vi "I(V)_K6221-K2182a_PK_fixedrange.vi"() -> ()   [LabVIEW 2016]
uses:
  Labview Drivers/Keithley 622x LV 2009/Configure/Source/Typedefs/KE622x -- Current Range.ctl
  Labview Drivers/Keithley 622x LV 2009/Configure/Source/Typedefs/KE622x -- Current Ranges.ctl
  Labview Drivers/Keithley 622x LV 2009/Keithley 622x.lvlib
panel:
  in  "Current Range In":T1
  out "Resistance (ohm)":dbl=inf format="%#_13g"
  out "Time (s)":dbl=95.61940909968689 format="%#_13g"
  in  "Total number of I-V loops":i32=1
  in  "Numeric Average":i32=1
  in  "wait (ms)":u32=50
  out "Iset (A)":dbl
  out "Vmeas (V)":dbl=1.84890386e-07
  in  "Folder":path=path "D:/Pranava/Data/PtTe2/31-05-2022/001/after warmup"
  in  "Set Compliance voltage (V)":dbl=20.0 min=0.0 step=0.1 format="%_3f"
  out "I vs V":cluster{dbl, "Field Reading":dbl}[](graph)=[{0.0, "Field Reading"=5.69524003e-09}, {1e-06, "Field Reading"=1.86435146e-08}, {2e-06, "Field Reading"=-1.55399303e-08}, {3e-06, "Field Reading"=5.69524003e-09}, {4e-06, "Field Reading"=1.03168822e-09}, {5e-06, "Field Reading"=-4.50641504e-08}, {6e-06, "Field Reading"=1.9677196e-08}, {7e-06, "Field Reading"=2.48565037e-08}, {8e-06, "Field Reading"=-4.71358735e-08}, {9e-06, "Field Reading"=3.52151191e-08}, {1e-05, "Field Reading"=1.08723729e-08}, {1.1e-05, "Field Reading"=1.34588038e-08}, {1.2e-05, "Field Reading"=-8.8122059e-09}, {1.3e-05, "Field Reading"=-8.8122059e-09}, {1.4e-05, "Field Reading"=3.00325784e-08}, {1.5e-05, "Field Reading"=1.08691515e-08}, {1.6e-05, "Field Reading"=3.10019462e-09}, {1.7e-05, "Field Reading"=-4.66876224e-09}, {1.8e-05, "Field Reading"=2.38174129e-08}, {1.9e-05, "Field Reading"=2.58874074e-08}, {2e-05, "Field Reading"=-2.90132033e-08}, {2.1e-05, "Field Reading"=-1.7618737e-08}, {2.2e-05, "Field Reading"=5.43735733e-08}, {2.3e-05, "Field Reading"=-3.05669942e-08}, {2.4e-05, "Field Reading"=4.76404796e-08}, {2.5e-05, "Field Reading"=-2.4869761e-08}, {2.6e-05, "Field Reading"=1.34592487e-08}, {2.7e-05, "Field Reading"=-5.70417987e-09}, {2.8e-05, "Field Reading"=-5.17999945e-08}, {2.9e-05, "Field Reading"=3.31406077e-08}, {3e-05, "Field Reading"=-3.41903574e-08}, {3.1e-05, "Field Reading"=4.29812872e-08}, {3.2e-05, "Field Reading"=2.17461367e-08}, {3.3e-05, "Field Reading"=1.54751787e-09}, {3.4e-05, "Field Reading"=-1.34724686e-08}, {3.5e-05, "Field Reading"=1.13881986e-08}, {3.6e-05, "Field Reading"=-4.19586497e-08}, {3.7e-05, "Field Reading"=2.27826711e-08}, {3.8e-05, "Field Reading"=-8.29316289e-09}, {3.9e-05, "Field Reading"=1.54751787e-09}, {4e-05, "Field Reading"=-5.70351006e-09}, {4.1e-05, "Field Reading"=-1.70968827e-08}, {4.2e-05, "Field Reading"=1.0353443e-08}, {4.3e-05, "Field Reading"=4.35010061e-08}, {4.4e-05, "Field Reading"=1.91582645e-08}, {4.5e-05, "Field Reading"=-3.05630803e-08}, {4.6e-05, "Field Reading"=-4.97265152e-08}, {4.7e-05, "Field Reading"=1.81224031e-08}, {4.8e-05, "Field Reading"=-2.64182465e-08}, {4.9e-05, "Field Reading"=-2.17568692e-08}, {5e-05, "Field Reading"=-2.17568692e-08}, {5.1e-05, "Field Reading"=-2.7972039e-08}, {5.2e-05, "Field Reading"=2.79644885e-08}, {5.3e-05, "Field Reading"=9.31897937e-09}, {5.4e-05, "Field Reading"=2.38210421e-08}, {5.5e-05, "Field Reading"=-1.0884604e-08}, {5.6e-05, "Field Reading"=4.24622263e-08}, {5.7e-05, "Field Reading"=3.09951655e-09}, {5.8e-05, "Field Reading"=-9.84874324e-09}, {5.9e-05, "Field Reading"=-4.14424971e-08}, {6e-05, "Field Reading"=4.8677391e-08}, {6.1e-05, "Field Reading"=6.11077204e-08}, {6.2e-05, "Field Reading"=1.13864028e-08}, {6.3e-05, "Field Reading"=-1.86539399e-08}, {6.4e-05, "Field Reading"=2.34902041e-05}, {6.5e-05, "Field Reading"=2.39584131e-05}, {6.6e-05, "Field Reading"=2.43251077e-05}, {6.7e-05, "Field Reading"=2.47192527e-05}, {6.8e-05, "Field Reading"=2.51320432e-05}, {6.9e-05, "Field Reading"=2.55598536e-05}, {7e-05, "Field Reading"=2.60389398e-05}, {7.1e-05, "Field Reading"=2.63802559e-05}, {7.2e-05, "Field Reading"=2.6751612e-05}, {7.3e-05, "Field Reading"=2.72110162e-05}, {7.4e-05, "Field Reading"=2.76004998e-05}, {7.5e-05, "Field Reading"=2.79930909e-05}, {7.6e-05, "Field Reading"=2.83862001e-05}, {7.7e-05, "Field Reading"=2.87430612e-05}, {7.8e-05, "Field Reading"=2.92268082e-05}, {7.9e-05, "Field Reading"=2.95531044e-05}, {8e-05, "Field Reading"=2.99746998e-05}, {8.1e-05, "Field Reading"=3.04107972e-05}, {8.2e-05, "Field Reading"=3.08132291e-05}, {8.3e-05, "Field Reading"=3.1164386e-05}, {8.4e-05, "Field Reading"=3.15694075e-05}, {8.5e-05, "Field Reading"=3.20283147e-05}, {8.6e-05, "Field Reading"=3.24348904e-05}, {8.7e-05, "Field Reading"=3.27865653e-05}, {8.8e-05, "Field Reading"=3.32169657e-05}, {8.9e-05, "Field Reading"=3.36380434e-05}, {9e-05, "Field Reading"=3.39819494e-05}, {9.1e-05, "Field Reading"=3.44465424e-05}, {9.2e-05, "Field Reading"=3.48645126e-05}, {9.3e-05, "Field Reading"=3.52482993e-05}, {9.4e-05, "Field Reading"=3.5625353e-05}, {9.5e-05, "Field Reading"=3.60288211e-05}, {9.6e-05, "Field Reading"=3.64131257e-05}, {9.7e-05, "Field Reading"=3.68409366e-05}, {9.8e-05, "Field Reading"=3.72257592e-05}, {9.9e-05, "Field Reading"=3.76105824e-05}, {0.0001, "Field Reading"=3.80508236e-05}, {0.000101, "Field Reading"=3.84517021e-05}, {0.000102, "Field Reading"=3.87945723e-05}, {0.000103, "Field Reading"=3.92016659e-05}, {0.000104, "Field Reading"=3.96232616e-05}, {0.000105, "Field Reading"=4.00904352e-05}, {0.000106, "Field Reading"=4.04229382e-05}, {0.000107, "Field Reading"=4.09087573e-05}, {0.000108, "Field Reading"=4.12573246e-05}, {0.000109, "Field Reading"=4.16566492e-05}, {0.00011, "Field Reading"=4.20709938e-05}, {0.000111, "Field Reading"=4.24951791e-05}, {0.000112, "Field Reading"=4.28644637e-05}, {0.000113, "Field Reading"=4.32772566e-05}, {0.000114, "Field Reading"=4.3693155e-05}, {0.000115, "Field Reading"=4.41230375e-05}, {0.000116, "Field Reading"=4.44912863e-05}, {0.000117, "Field Reading"=4.4905113e-05}, {0.000118, "Field Reading"=4.53142783e-05}, {0.000119, "Field Reading"=4.57451966e-05}, {0.00012, "Field Reading"=4.61693819e-05}, {0.000121, "Field Reading"=4.65593711e-05}, {0.000122, "Field Reading"=4.69462653e-05}, {0.000123, "Field Reading"=4.74134387e-05}, {0.000124, "Field Reading"=4.78179425e-05}, {0.000125, "Field Reading"=4.81789402e-05}, {0.000126, "Field Reading"=4.86310936e-05}, {0.000127, "Field Reading"=4.90894622e-05}, {0.000128, "Field Reading"=4.94913942e-05}, {0.000129, "Field Reading"=4.98182085e-05}, {0.00013, "Field Reading"=5.02667366e-05}, {0.000131, "Field Reading"=5.07411612e-05}, {0.000132, "Field Reading"=5.11741513e-05}, {0.000133, "Field Reading"=5.15320415e-05}, {0.000134, "Field Reading"=5.1924633e-05}, {0.000135, "Field Reading"=5.22545517e-05}, {0.000136, "Field Reading"=5.27786976e-05}, {0.000137, "Field Reading"=5.32028829e-05}, {0.000138, "Field Reading"=5.35498965e-05}, {0.000139, "Field Reading"=5.39668308e-05}, {0.00014, "Field Reading"=5.44692236e-05}, {0.000141, "Field Reading"=5.47851614e-05}, {0.000142, "Field Reading"=5.52129722e-05}, {0.000143, "Field Reading"=5.56153793e-05}, {0.000144, "Field Reading"=5.60509589e-05}, {0.000145, "Field Reading"=5.64575344e-05}, {0.000146, "Field Reading"=5.68423568e-05}, {0.000147, "Field Reading"=5.7332837e-05}, {0.000148, "Field Reading"=5.77010856e-05}, {0.000149, "Field Reading"=5.80838363e-05}, {0.00015, "Field Reading"=5.85660081e-05}, {0.00015, "Field Reading"=5.85986377e-05}, {0.000149, "Field Reading"=5.80952094e-05}, {0.000148, "Field Reading"=5.767465e-05}, {0.000147, "Field Reading"=5.73058836e-05}, {0.000146, "Field Reading"=5.68801448e-05}, {0.000145, "Field Reading"=5.65103425e-05}, {0.000144, "Field Reading"=5.60778901e-05}, {0.000143, "Field Reading"=5.56329878e-05}, {0.000142, "Field Reading"=5.52310737e-05}, {0.000141, "Field Reading"=5.48478051e-05}, {0.00014, "Field Reading"=5.43966876e-05}, {0.000139, "Field Reading"=5.39958094e-05}, {0.000138, "Field Reading"=5.36083974e-05}, {0.000137, "Field Reading"=5.31334551e-05}, {0.000136, "Field Reading"=5.27263627e-05}, {0.000135, "Field Reading"=5.23539706e-05}, {0.000134, "Field Reading"=5.19701841e-05}, {0.000133, "Field Reading"=5.15102618e-05}, {0.000132, "Field Reading"=5.10767539e-05}, {0.000131, "Field Reading"=5.06815729e-05}, {0.00013, "Field Reading"=5.03112526e-05}, {0.000129, "Field Reading"=4.99316069e-05}, {0.000128, "Field Reading"=4.95022425e-05}, {0.000127, "Field Reading"=4.90236747e-05}, {0.000126, "Field Reading"=4.86590516e-05}, {0.000125, "Field Reading"=4.8298054e-05}, {0.000124, "Field Reading"=4.78526338e-05}, {0.000123, "Field Reading"=4.74331101e-05}, {0.000122, "Field Reading"=4.70338163e-05}, {0.000121, "Field Reading"=4.66567626e-05}, {0.00012, "Field Reading"=4.62491511e-05}, {0.000119, "Field Reading"=4.58311809e-05}, {0.000118, "Field Reading"=4.54318562e-05}, {0.000117, "Field Reading"=4.50506591e-05}, {0.000116, "Field Reading"=4.45938441e-05}, {0.000115, "Field Reading"=4.41727664e-05}, {0.000114, "Field Reading"=4.37987887e-05}, {0.000113, "Field Reading"=4.34227711e-05}, {0.000112, "Field Reading"=4.29882274e-05}, {0.000111, "Field Reading"=4.25780265e-05}, {0.00011, "Field Reading"=4.22341206e-05}, {0.000109, "Field Reading"=4.18316886e-05}, {0.000108, "Field Reading"=4.13986987e-05}, {0.000107, "Field Reading"=4.09154706e-05}, {0.000106, "Field Reading"=4.05446324e-05}, {0.000105, "Field Reading"=4.01655073e-05}, {0.000104, "Field Reading"=3.97755056e-05}, {0.000103, "Field Reading"=3.94046673e-05}, {0.000102, "Field Reading"=3.89846257e-05}, {0.000101, "Field Reading"=3.85687275e-05}, {0.0001, "Field Reading"=3.81668178e-05}, {9.9e-05, "Field Reading"=3.77840672e-05}, {9.8e-05, "Field Reading"=3.73800813e-05}, {9.7e-05, "Field Reading"=3.6964701e-05}, {9.6e-05, "Field Reading"=3.65876475e-05}, {9.5e-05, "Field Reading"=3.61862513e-05}, {9.4e-05, "Field Reading"=3.57418669e-05}, {9.3e-05, "Field Reading"=3.54010586e-05}, {9.2e-05, "Field Reading"=3.49520129e-05}, {9.1e-05, "Field Reading"=3.45050389e-05}, {9e-05, "Field Reading"=3.41409338e-05}, {8.9e-05, "Field Reading"=3.37934025e-05}, {8.8e-05, "Field Reading"=3.33686995e-05}, {8.7e-05, "Field Reading"=3.2970411e-05}, {8.6e-05, "Field Reading"=3.2593365e-05}, {8.5e-05, "Field Reading"=3.22489412e-05}, {8.4e-05, "Field Reading"=3.17481023e-05}, {8.3e-05, "Field Reading"=3.14010889e-05}, {8.2e-05, "Field Reading"=3.09567045e-05}, {8.1e-05, "Field Reading"=3.05817227e-05}, {8e-05, "Field Reading"=3.01492507e-05}, {7.9e-05, "Field Reading"=2.97685718e-05}, {7.8e-05, "Field Reading"=2.93438618e-05}, {7.7e-05, "Field Reading"=2.90129043e-05}, {7.6e-05, "Field Reading"=2.85358903e-05}, {7.5e-05, "Field Reading"=2.81464066e-05}, {7.4e-05, "Field Reading"=2.78107877e-05}, {7.3e-05, "Field Reading"=2.73721006e-05}, {7.2e-05, "Field Reading"=2.69810631e-05}, {7.1e-05, "Field Reading"=2.6545994e-05}, {7e-05, "Field Reading"=2.61259525e-05}, {6.9e-05, "Field Reading"=2.5727664e-05}, {6.8e-05, "Field Reading"=2.54143162e-05}, {6.7e-05, "Field Reading"=2.49150313e-05}, {6.6e-05, "Field Reading"=2.45364243e-05}, {6.5e-05, "Field Reading"=2.41101676e-05}, {6.4e-05, "Field Reading"=2.37274173e-05}, {6.3e-05, "Field Reading"=2.32561007e-05}, {6.2e-05, "Field Reading"=2.28702426e-05}, {6.1e-05, "Field Reading"=2.24574521e-05}, {6e-05, "Field Reading"=2.20229085e-05}, {5.9e-05, "Field Reading"=2.15950981e-05}, {5.8e-05, "Field Reading"=2.11512318e-05}, {5.7e-05, "Field Reading"=2.07586406e-05}, {5.6e-05, "Field Reading"=2.03329035e-05}, {5.5e-05, "Field Reading"=1.98952523e-05}, {5.4e-05, "Field Reading"=1.94612267e-05}, {5.3e-05, "Field Reading"=1.90038942e-05}, {5.2e-05, "Field Reading"=1.8551223e-05}, {5.1e-05, "Field Reading"=1.80809422e-05}, {5e-05, "Field Reading"=1.76241276e-05}, {4.9e-05, "Field Reading"=1.71724962e-05}, {4.8e-05, "Field Reading"=1.66587092e-05}, {4.7e-05, "Field Reading"=1.61713366e-05}, {4.6e-05, "Field Reading"=1.56368323e-05}, {4.5e-05, "Field Reading"=1.51396191e-05}, {4.4e-05, "Field Reading"=1.45895769e-05}, {4.3e-05, "Field Reading"=1.40100127e-05}, {4.2e-05, "Field Reading"=1.33589784e-05}, {4.1e-05, "Field Reading"=1.27302107e-05}, {4e-05, "Field Reading"=1.20978174e-05}, {3.9e-05, "Field Reading"=1.13219574e-05}, {3.8e-05, "Field Reading"=1.03239051e-05}, {3.7e-05, "Field Reading"=9.26473704e-06}, {3.6e-05, "Field Reading"=2.63103012e-07}, {3.5e-05, "Field Reading"=2.08202367e-07}, {3.4e-05, "Field Reading"=2.38242436e-07}, {3.3e-05, "Field Reading"=2.5015484e-07}, {3.2e-05, "Field Reading"=2.13899697e-07}, {3.1e-05, "Field Reading"=2.51708632e-07}, {3e-05, "Field Reading"=1.90074888e-07}, {2.9e-05, "Field Reading"=2.22704517e-07}, {2.8e-05, "Field Reading"=2.64656898e-07}, {2.7e-05, "Field Reading"=2.52744229e-07}, {2.6e-05, "Field Reading"=2.12863572e-07}, {2.5e-05, "Field Reading"=2.82784203e-07}, {2.4e-05, "Field Reading"=1.75054638e-07}, {2.3e-05, "Field Reading"=1.94736001e-07}, {2.2e-05, "Field Reading"=2.50672506e-07}, {2.1e-05, "Field Reading"=2.7138973e-07}, {2e-05, "Field Reading"=2.04059697e-07}, {1.9e-05, "Field Reading"=2.51709321e-07}, {1.8e-05, "Field Reading"=2.38761053e-07}, {1.7e-05, "Field Reading"=2.59478281e-07}, {1.6e-05, "Field Reading"=2.56888628e-07}, {1.5e-05, "Field Reading"=2.2840244e-07}, {1.4e-05, "Field Reading"=2.49637598e-07}, {1.3e-05, "Field Reading"=2.20633479e-07}, {1.2e-05, "Field Reading"=2.58959681e-07}, {1.1e-05, "Field Reading"=2.42903832e-07}, {1e-05, "Field Reading"=2.14417647e-07}, {9e-06, "Field Reading"=2.65174849e-07}, {8e-06, "Field Reading"=2.54816236e-07}, {7e-06, "Field Reading"=2.00951451e-07}, {6e-06, "Field Reading"=2.05612827e-07}, {5e-06, "Field Reading"=1.86967902e-07}, {4e-06, "Field Reading"=2.04577545e-07}, {3e-06, "Field Reading"=2.55852683e-07}, {2e-06, "Field Reading"=2.0820306e-07}, {1e-06, "Field Reading"=2.29438218e-07}, {0.0, "Field Reading"=2.43422347e-07}, {-1e-06, "Field Reading"=2.27366495e-07}, {-2e-06, "Field Reading"=2.22704088e-07}, {-3e-06, "Field Reading"=2.25811672e-07}, {-4e-06, "Field Reading"=1.83859294e-07}, {-5e-06, "Field Reading"=1.77644127e-07}, {-6e-06, "Field Reading"=1.77126197e-07}, {-7e-06, "Field Reading"=2.26329603e-07}, {-8e-06, "Field Reading"=1.47086223e-07}, {-9e-06, "Field Reading"=2.51190271e-07}, {-1e-05, "Field Reading"=1.78679016e-07}, {-1.1e-05, "Field Reading"=1.84376252e-07}, {-1.2e-05, "Field Reading"=2.25292761e-07}, {-1.3e-05, "Field Reading"=1.64694893e-07}, {-1.4e-05, "Field Reading"=1.83340391e-07}, {-1.5e-05, "Field Reading"=2.27882413e-07}, {-1.6e-05, "Field Reading"=1.83340391e-07}, {-1.7e-05, "Field Reading"=1.49155896e-07}, {-1.8e-05, "Field Reading"=1.5485313e-07}, {-1.9e-05, "Field Reading"=1.75570346e-07}, {-2e-05, "Field Reading"=1.76606206e-07}, {-2.1e-05, "Field Reading"=2.01466865e-07}, {-2.2e-05, "Field Reading"=2.15450986e-07}, {-2.3e-05, "Field Reading"=1.64693807e-07}, {-2.4e-05, "Field Reading"=1.49155719e-07}, {-2.5e-05, "Field Reading"=1.79195681e-07}, {-2.6e-05, "Field Reading"=1.71944656e-07}, {-2.7e-05, "Field Reading"=1.51227441e-07}, {-2.8e-05, "Field Reading"=1.56924675e-07}, {-2.9e-05, "Field Reading"=1.57960536e-07}, {-3e-05, "Field Reading"=7.25020236e-08}, {-3.1e-05, "Field Reading"=1.56924675e-07}, {-3.2e-05, "Field Reading"=1.41904071e-07}, {-3.3e-05, "Field Reading"=1.60031632e-07}, {-3.4e-05, "Field Reading"=1.98358476e-07}, {-3.5e-05, "Field Reading"=1.3931442e-07}, {-3.6e-05, "Field Reading"=1.42939932e-07}, {-3.7e-05, "Field Reading"=1.16007555e-07}, {-3.8e-05, "Field Reading"=1.2429444e-07}, {-3.9e-05, "Field Reading"=1.28954276e-07}, {-4e-05, "Field Reading"=1.57958365e-07}, {-4.1e-05, "Field Reading"=1.27918415e-07}, {-4.2e-05, "Field Reading"=1.56922505e-07}, {-4.3e-05, "Field Reading"=1.52779064e-07}, {-4.4e-05, "Field Reading"=1.30508066e-07}, {-4.5e-05, "Field Reading"=8.75198623e-08}, {-4.6e-05, "Field Reading"=1.54850399e-07}, {-4.7e-05, "Field Reading"=8.95912018e-08}, {-4.8e-05, "Field Reading"=1.13415988e-07}, {-4.9e-05, "Field Reading"=1.11344267e-07}, {-5e-05, "Field Reading"=1.09272547e-07}, {-5.1e-05, "Field Reading"=1.08754617e-07}, {-5.2e-05, "Field Reading"=1.01503595e-07}, {-5.3e-05, "Field Reading"=6.68022759e-08}, {-5.4e-05, "Field Reading"=1.06682209e-07}, {-5.5e-05, "Field Reading"=5.85147131e-08}, {-5.6e-05, "Field Reading"=8.95905172e-08}, {-5.7e-05, "Field Reading"=6.31760837e-08}, {-5.8e-05, "Field Reading"=7.81960557e-08}, {-5.9e-05, "Field Reading"=8.23394962e-08}, {-6e-05, "Field Reading"=7.09450347e-08}, {-6.1e-05, "Field Reading"=6.26585952e-08}, {-6.2e-05, "Field Reading"=8.18220093e-08}, {-6.3e-05, "Field Reading"=1.22738488e-07}, {-6.4e-05, "Field Reading"=8.54475201e-08}, {-6.5e-05, "Field Reading"=1.00985423e-07}, {-6.6e-05, "Field Reading"=3.05469284e-08}, {-6.7e-05, "Field Reading"=8.07861491e-08}, {-6.8e-05, "Field Reading"=5.85159761e-08}, {-6.9e-05, "Field Reading"=6.05876968e-08}, {-7e-05, "Field Reading"=5.69621855e-08}, {-7.1e-05, "Field Reading"=3.21015364e-08}, {-7.2e-05, "Field Reading"=4.91932327e-08}, {-7.3e-05, "Field Reading"=-2.70042176e-05}, {-7.4e-05, "Field Reading"=-2.73548538e-05}, {-7.5e-05, "Field Reading"=-2.78168443e-05}, {-7.6e-05, "Field Reading"=-2.82348164e-05}, {-7.7e-05, "Field Reading"=-2.86305123e-05}, {-7.8e-05, "Field Reading"=-2.9042264e-05}, {-7.9e-05, "Field Reading"=-2.94431392e-05}, {-8e-05, "Field Reading"=-2.99046118e-05}, {-8.1e-05, "Field Reading"=-3.02707859e-05}, {-8.2e-05, "Field Reading"=-3.06711432e-05}, {-8.3e-05, "Field Reading"=-3.10538902e-05}, {-8.4e-05, "Field Reading"=-3.1429387e-05}, {-8.5e-05, "Field Reading"=-3.18442462e-05}, {-8.6e-05, "Field Reading"=-3.2276197e-05}, {-8.7e-05, "Field Reading"=-3.26791439e-05}, {-8.8e-05, "Field Reading"=-3.30748398e-05}, {-8.9e-05, "Field Reading"=-3.34394602e-05}, {-9e-05, "Field Reading"=-3.38584657e-05}, {-9.1e-05, "Field Reading"=-3.43064722e-05}, {-9.2e-05, "Field Reading"=-3.4654001e-05}, {-9.3e-05, "Field Reading"=-3.51367086e-05}, {-9.4e-05, "Field Reading"=-3.54754327e-05}, {-9.5e-05, "Field Reading"=-3.59011684e-05}, {-9.6e-05, "Field Reading"=-3.62507689e-05}, {-9.7e-05, "Field Reading"=-3.66563054e-05}, {-9.8e-05, "Field Reading"=-3.71224399e-05}, {-9.9e-05, "Field Reading"=-3.75471398e-05}, {-0.0001, "Field Reading"=-3.79050271e-05}, {-0.000101, "Field Reading"=-3.82365002e-05}, {-0.000102, "Field Reading"=-3.87083314e-05}, {-0.000103, "Field Reading"=-3.91076528e-05}, {-0.000104, "Field Reading"=-3.9509046e-05}, {-0.000105, "Field Reading"=-3.98690135e-05}, {-0.000106, "Field Reading"=-4.03258249e-05}, {-0.000107, "Field Reading"=-4.0721003e-05}, {-0.000108, "Field Reading"=-4.10856235e-05}, {-0.000109, "Field Reading"=-4.14916781e-05}, {-0.00011, "Field Reading"=-4.18780515e-05}, {-0.000111, "Field Reading"=-4.235558e-05}, {-0.000112, "Field Reading"=-4.27093295e-05}, {-0.000113, "Field Reading"=-4.31112408e-05}, {-0.000114, "Field Reading"=-4.35328332e-05}, {-0.000115, "Field Reading"=-4.406578e-05}, {-0.000116, "Field Reading"=-4.43635879e-05}, {-0.000117, "Field Reading"=-4.4724065e-05}, {-0.000118, "Field Reading"=-4.51539443e-05}, {-0.000119, "Field Reading"=-4.55605169e-05}, {-0.00012, "Field Reading"=-4.59686458e-05}, {-0.000121, "Field Reading"=-4.63389636e-05}, {-0.000122, "Field Reading"=-4.67320701e-05}, {-0.000123, "Field Reading"=-4.7228762e-05}, {-0.000124, "Field Reading"=-4.75421078e-05}, {-0.000125, "Field Reading"=-4.79906325e-05}, {-0.000126, "Field Reading"=-4.84293165e-05}, {-0.000127, "Field Reading"=-4.88897812e-05}, {-0.000128, "Field Reading"=-4.92481868e-05}, {-0.000129, "Field Reading"=-4.95838037e-05}, {-0.00013, "Field Reading"=-5.0108464e-05}, {-0.000131, "Field Reading"=-5.05362719e-05}, {-0.000132, "Field Reading"=-5.08848369e-05}, {-0.000133, "Field Reading"=-5.13442383e-05}, {-0.000134, "Field Reading"=-5.17606354e-05}, {-0.000135, "Field Reading"=-5.21848176e-05}, {-0.000136, "Field Reading"=-5.25577251e-05}, {-0.000137, "Field Reading"=-5.29461704e-05}, {-0.000138, "Field Reading"=-5.34402728e-05}, {-0.000139, "Field Reading"=-5.384322e-05}, {-0.00014, "Field Reading"=-5.42358087e-05}, {-0.000141, "Field Reading"=-5.46361663e-05}, {-0.000142, "Field Reading"=-5.50287621e-05}, {-0.000143, "Field Reading"=-5.54425859e-05}, {-0.000144, "Field Reading"=-5.58911107e-05}, {-0.000145, "Field Reading"=-5.62971656e-05}, {-0.000146, "Field Reading"=-5.66825034e-05}, {-0.000147, "Field Reading"=-5.70911479e-05}, {-0.000148, "Field Reading"=-5.75852503e-05}, {-0.000149, "Field Reading"=-5.79835108e-05}, {-0.00015, "Field Reading"=-5.83781711e-05}, {-0.00015, "Field Reading"=-5.838594e-05}, {-0.000149, "Field Reading"=-5.79011605e-05}, {-0.000148, "Field Reading"=-5.75531136e-05}, {-0.000147, "Field Reading"=-5.71278956e-05}, {-0.000146, "Field Reading"=-5.67151079e-05}, {-0.000145, "Field Reading"=-5.62785034e-05}, {-0.000144, "Field Reading"=-5.58755562e-05}, {-0.000143, "Field Reading"=-5.55026488e-05}, {-0.000142, "Field Reading"=-5.50251202e-05}, {-0.000141, "Field Reading"=-5.45978305e-05}, {-0.00014, "Field Reading"=-5.42218155e-05}, {-0.000139, "Field Reading"=-5.38732507e-05}, {-0.000138, "Field Reading"=-5.34200646e-05}, {-0.000137, "Field Reading"=-5.30052245e-05}, {-0.000136, "Field Reading"=-5.25556637e-05}, {-0.000135, "Field Reading"=-5.21252663e-05}, {-0.000134, "Field Reading"=-5.18450677e-05}, {-0.000133, "Field Reading"=-5.13841125e-05}, {-0.000132, "Field Reading"=-5.0961484e-05}, {-0.000131, "Field Reading"=-5.052021e-05}, {-0.00013, "Field Reading"=-5.00784318e-05}, {-0.000129, "Field Reading"=-4.97324564e-05}, {-0.000128, "Field Reading"=-4.93486723e-05}, {-0.000127, "Field Reading"=-4.89193105e-05}, {-0.000126, "Field Reading"=-4.84443712e-05}, {-0.000125, "Field Reading"=-4.80683559e-05}, {-0.000124, "Field Reading"=-4.76540141e-05}, {-0.000123, "Field Reading"=-4.72272693e-05}, {-0.000122, "Field Reading"=-4.68082658e-05}, {-0.000121, "Field Reading"=-4.64441627e-05}, {-0.00012, "Field Reading"=-4.60463942e-05}, {-0.000119, "Field Reading"=-4.56263549e-05}, {-0.000118, "Field Reading"=-4.51767937e-05}, {-0.000117, "Field Reading"=-4.48282284e-05}, {-0.000116, "Field Reading"=-4.43460377e-05}, {-0.000115, "Field Reading"=-4.39544663e-05}, {-0.000114, "Field Reading"=-4.35934709e-05}, {-0.000113, "Field Reading"=-4.31185315e-05}, {-0.000112, "Field Reading"=-4.27647871e-05}, {-0.000111, "Field Reading"=-4.23317998e-05}, {-0.00011, "Field Reading"=-4.19780553e-05}, {-0.000109, "Field Reading"=-4.15341915e-05}, {-0.000108, "Field Reading"=-4.1154029e-05}, {-0.000107, "Field Reading"=-4.07780138e-05}, {-0.000106, "Field Reading"=-4.03786918e-05}, {-0.000105, "Field Reading"=-3.9935346e-05}, {-0.000104, "Field Reading"=-3.94712831e-05}, {-0.000103, "Field Reading"=-3.91227179e-05}, {-0.000102, "Field Reading"=-3.87202884e-05}, {-0.000101, "Field Reading"=-3.83250902e-05}, {-0.0001, "Field Reading"=-3.78708681e-05}, {-9.9e-05, "Field Reading"=-3.74694747e-05}, {-9.8e-05, "Field Reading"=-3.70774039e-05}, {-9.7e-05, "Field Reading"=-3.67495561e-05}, {-9.6e-05, "Field Reading"=-3.62368083e-05}, {-9.5e-05, "Field Reading"=-3.58670084e-05}, {-9.4e-05, "Field Reading"=-3.54557743e-05}, {-9.3e-05, "Field Reading"=-3.50958001e-05}, {-9.2e-05, "Field Reading"=-3.46534907e-05}, {-9.1e-05, "Field Reading"=-3.4275922e-05}, {-9e-05, "Field Reading"=-3.38620985e-05}, {-8.9e-05, "Field Reading"=-3.3497996e-05}, {-8.8e-05, "Field Reading"=-3.30499893e-05}, {-8.7e-05, "Field Reading"=-3.26672414e-05}, {-8.6e-05, "Field Reading"=-3.22912106e-05}, {-8.5e-05, "Field Reading"=-3.18121286e-05}, {-8.4e-05, "Field Reading"=-3.14174686e-05}, {-8.3e-05, "Field Reading"=-3.10476691e-05}, {-8.2e-05, "Field Reading"=-3.06545629e-05}, {-8.1e-05, "Field Reading"=-3.0259385e-05}, {-8e-05, "Field Reading"=-2.98538486e-05}, {-7.9e-05, "Field Reading"=-2.94296646e-05}, {-7.8e-05, "Field Reading"=-2.90142876e-05}, {-7.7e-05, "Field Reading"=-2.86092691e-05}, {-7.6e-05, "Field Reading"=-2.82358441e-05}, {-7.5e-05, "Field Reading"=-2.77759255e-05}, {-7.4e-05, "Field Reading"=-2.74019826e-05}, {-7.3e-05, "Field Reading"=-2.69814263e-05}, {-7.2e-05, "Field Reading"=-2.65919456e-05}, {-7.1e-05, "Field Reading"=-2.61522416e-05}, {-7e-05, "Field Reading"=-2.57560276e-05}, {-6.9e-05, "Field Reading"=-2.534324e-05}, {-6.8e-05, "Field Reading"=-2.49164682e-05}, {-6.7e-05, "Field Reading"=-2.4514557e-05}, {-6.6e-05, "Field Reading"=-2.41022873e-05}, {-6.5e-05, "Field Reading"=-2.36314918e-05}, {-6.4e-05, "Field Reading"=-2.32176717e-05}, {-6.3e-05, "Field Reading"=-2.28338879e-05}, {-6.2e-05, "Field Reading"=-2.23553234e-05}, {-6.1e-05, "Field Reading"=-2.19026553e-05}, {-6e-05, "Field Reading"=-2.15095487e-05}, {-5.9e-05, "Field Reading"=-2.10625778e-05}, {-5.8e-05, "Field Reading"=-2.05643321e-05}, {-5.7e-05, "Field Reading"=-2.01893601e-05}, {-5.6e-05, "Field Reading"=-1.9727369e-05}, {-5.5e-05, "Field Reading"=-1.92182466e-05}, {-5.4e-05, "Field Reading"=-1.87666141e-05}, {-5.3e-05, "Field Reading"=-1.82398822e-05}, {-5.2e-05, "Field Reading"=-1.77980903e-05}, {-5.1e-05, "Field Reading"=-1.72630716e-05}, {-5e-05, "Field Reading"=-1.66881747e-05}, {-4.9e-05, "Field Reading"=-1.62008051e-05}, {-4.8e-05, "Field Reading"=-1.55984557e-05}, {-4.7e-05, "Field Reading"=-1.50287357e-05}, {-4.6e-05, "Field Reading"=-1.44678205e-05}, {-4.5e-05, "Field Reading"=-1.37753517e-05}, {-4.4e-05, "Field Reading"=-1.3046628e-05}, {-4.3e-05, "Field Reading"=-1.23536368e-05}, {-4.2e-05, "Field Reading"=-1.14394958e-05}, {-4.1e-05, "Field Reading"=-1.02741601e-05}, {-4e-05, "Field Reading"=1.13939122e-07}, {-3.9e-05, "Field Reading"=6.62895039e-08}, {-3.8e-05, "Field Reading"=1.02544648e-07}, {-3.7e-05, "Field Reading"=1.42943237e-07}, {-3.6e-05, "Field Reading"=1.12903261e-07}, {-3.5e-05, "Field Reading"=9.06307346e-08}, {-3.4e-05, "Field Reading"=1.55372045e-07}, {-3.3e-05, "Field Reading"=1.61587211e-07}, {-3.2e-05, "Field Reading"=1.47603088e-07}, {-3.1e-05, "Field Reading"=1.51746532e-07}, {-3e-05, "Field Reading"=2.28400244e-07}, {-2.9e-05, "Field Reading"=1.37244478e-07}, {-2.8e-05, "Field Reading"=1.82823236e-07}, {-2.7e-05, "Field Reading"=1.83859097e-07}, {-2.6e-05, "Field Reading"=1.34137763e-07}, {-2.5e-05, "Field Reading"=1.67285319e-07}, {-2.4e-05, "Field Reading"=1.10830887e-07}, {-2.3e-05, "Field Reading"=1.56926708e-07}, {-2.2e-05, "Field Reading"=2.20632168e-07}, {-2.1e-05, "Field Reading"=1.96801734e-07}, {-2e-05, "Field Reading"=1.21701878e-07}, {-1.9e-05, "Field Reading"=1.65725932e-07}, {-1.8e-05, "Field Reading"=2.20108586e-07}, {-1.7e-05, "Field Reading"=2.02498964e-07}, {-1.6e-05, "Field Reading"=1.23255668e-07}, {-1.5e-05, "Field Reading"=1.79192113e-07}, {-1.4e-05, "Field Reading"=1.71941092e-07}, {-1.3e-05, "Field Reading"=2.02500563e-07}, {-1.2e-05, "Field Reading"=2.36166025e-07}, {-1.1e-05, "Field Reading"=2.16484678e-07}, {-1e-05, "Field Reading"=2.16484678e-07}, {-9e-06, "Field Reading"=1.80229565e-07}, {-8e-06, "Field Reading"=1.81783356e-07}, {-7e-06, "Field Reading"=2.43417048e-07}, {-6e-06, "Field Reading"=1.2273877e-07}, {-5e-06, "Field Reading"=2.04571731e-07}, {-4e-06, "Field Reading"=1.80746945e-07}, {-3e-06, "Field Reading"=1.74531783e-07}, {-2e-06, "Field Reading"=1.95766919e-07}, {-1e-06, "Field Reading"=2.11822753e-07}, {0.0, "Field Reading"=1.84890386e-07}]
  out "data":dbl[](array[numeric])=[1.84890386e-07, 0.0, inf]
  in  "Nanovoltmeter 2182a VISA":refnum<visa-resource-name>="GPIB0::7::INSTR"
  in  "Current source K6221 VISA":refnum<visa-resource-name>="GPIB0::12::INSTR"
  in  "Step":dbl[](array[numeric])=[1e-06, 1e-06, 1e-06] min=-3000.0 max=3000.0 format="%.1e"
  in  "To":dbl[](array[numeric])=[0.00015, -0.00015, 0.0] min=-3000.0 max=3000.0 format="%.1e"
  in  "From":dbl[](array[numeric])=[0.0, 0.00015, -0.00015] min=-3000.0 max=3000.0 format="%.1e"
  in  "file name":string="028_31-05-2022_001_DevB1_DC_IV_baseT_ZFC_afterwarmup"
  out "File path":path=path "D:/Pranava/Data/PtTe2/31-05-2022/001/after warmup/028_31-05-2022_001_DevB1_DC_IV_baseT_ZFC_afterwarmup.dat"
  # ".dat"
  # "Set Current (A)"
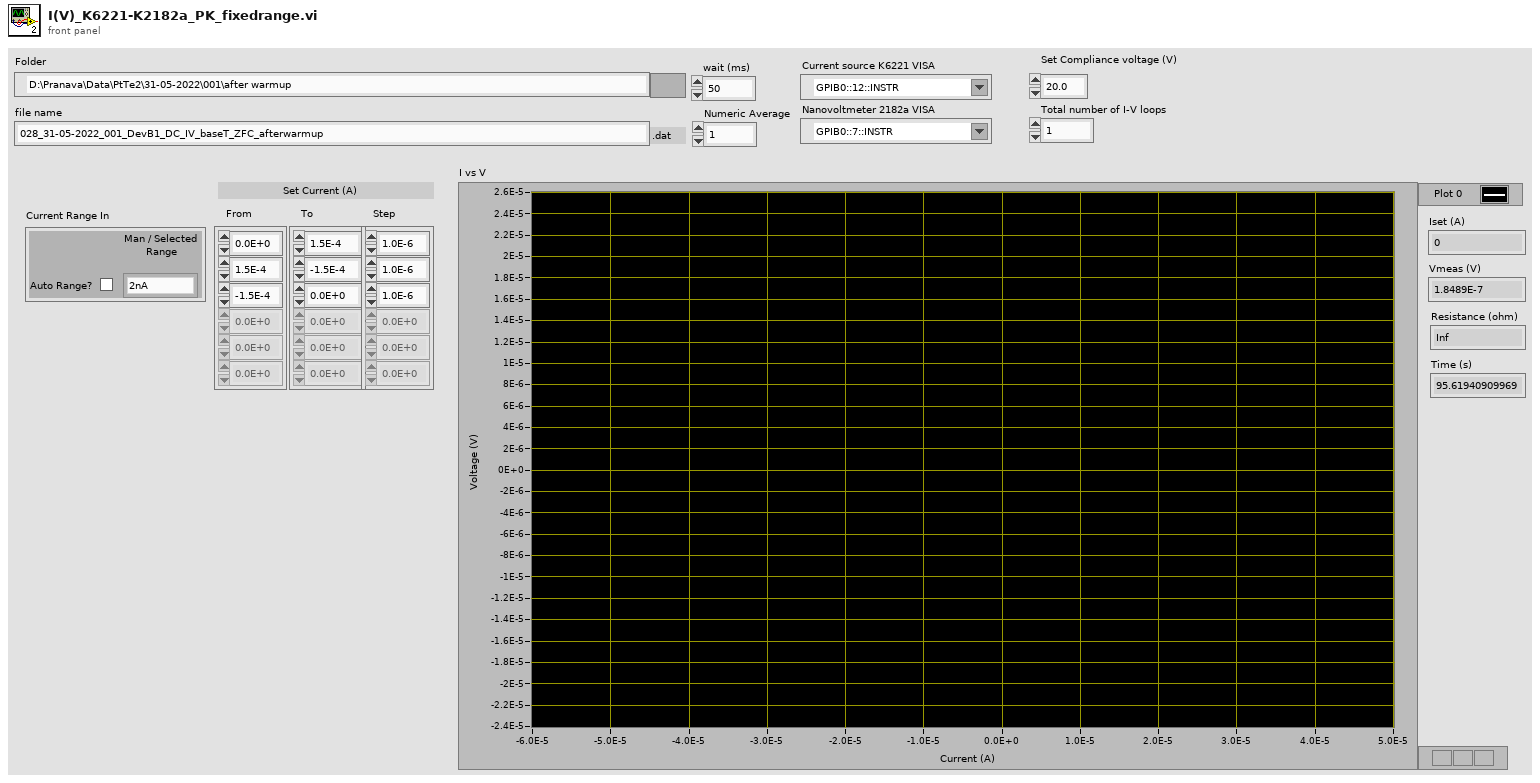
[diagram p1: front panel]
types:
  T1 = typedef "Keithley 622x.lvlib/KE622x -- Current Range.ctl" = cluster{"Auto Range?":bool, "Man / Selected\nRange":T2}
  T2 = typedef "Keithley 622x.lvlib/KE622x -- Current Ranges.ctl" = enum16{"2nA", "20nA", "200nA", "2uA", "20uA", "200uA", "2mA", "20mA", "100mA"}
  T3 = enum16{"open", "replace", "create", "open or create", "replace or create", "replace or create with confirmation"}
  T4 = typedef "Keithley 622x.lvlib/KE622x -- Current Level.ctl" = dbl
  T5 = cluster{"Average value":dbl, "Average value":dbl}
  T6 = cluster{"Average value":dbl, "Average value":dbl}[]
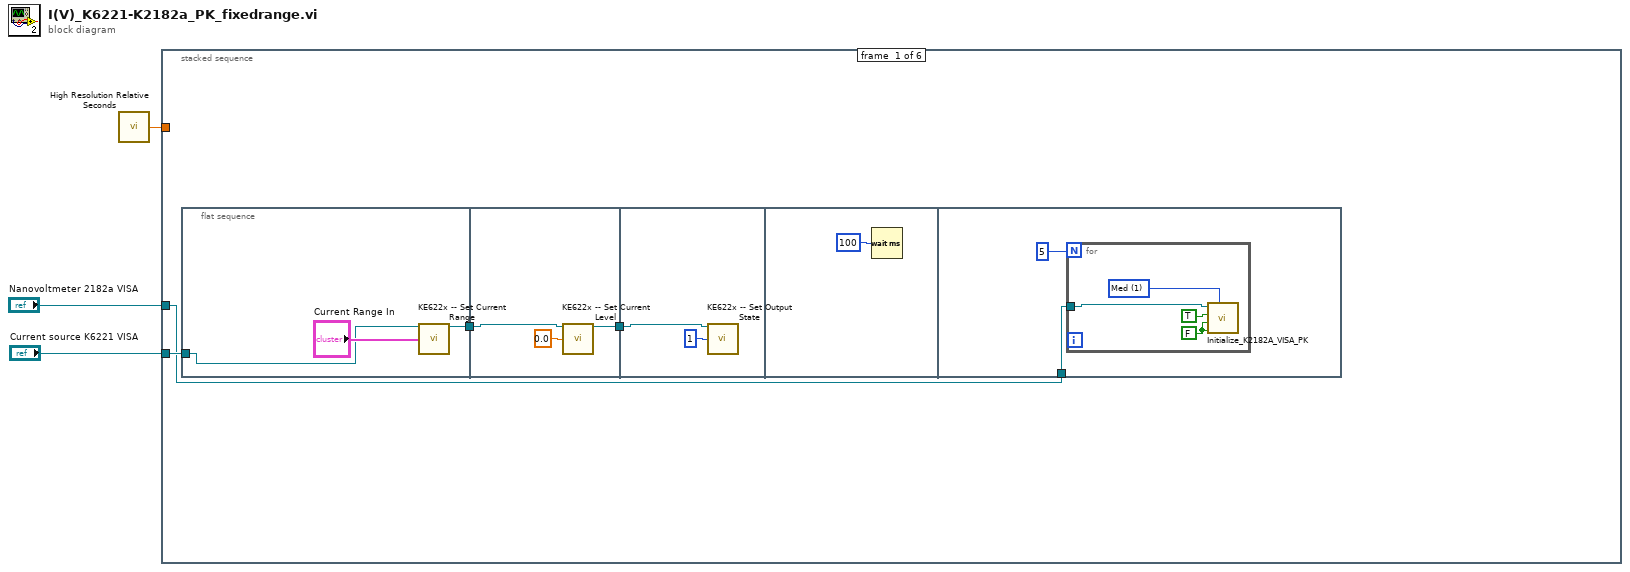
[diagram p0: block diagram]
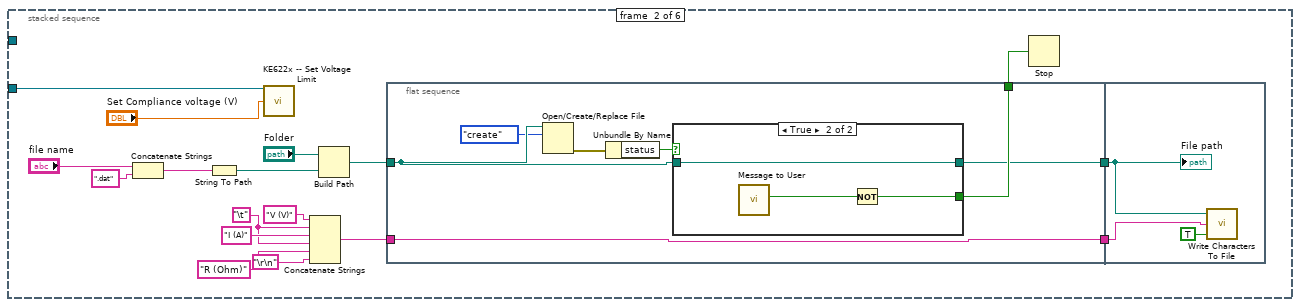
[diagram p2: hidden frame]
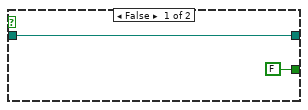
[diagram p3: hidden frame]
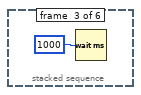
[diagram p4: hidden frame]
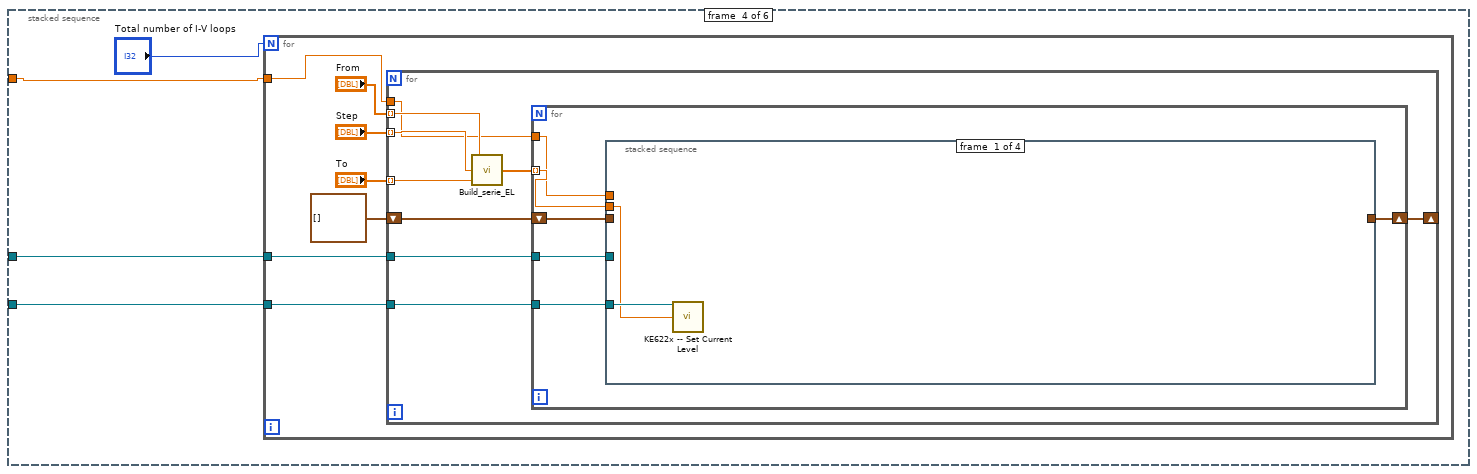
[diagram p5: hidden frame]
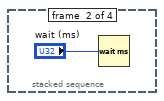
[diagram p6: hidden frame]
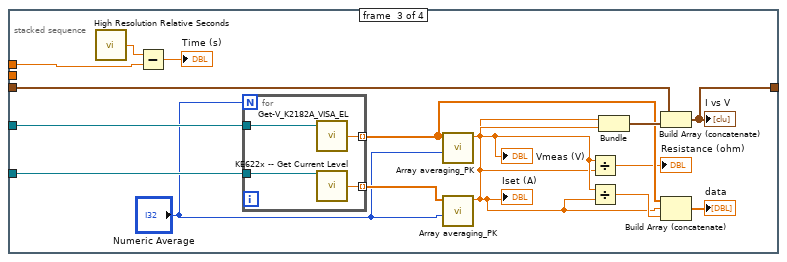
[diagram p7: hidden frame]
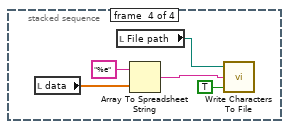
[diagram p8: hidden frame]
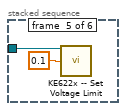
[diagram p9: hidden frame]
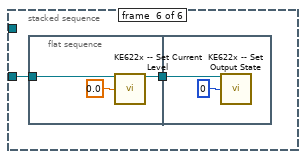
[diagram p10: hidden frame]
diagram:
  n1 = call <vilib>:"High Resolution Relative Seconds.vi"() -> ("relative seconds"=w1:dbl)
  n2 = stacked-sequence {
    tunnel: "Nanovoltmeter 2182a VISA" -> [w5 _ _ w59 _ _]
    tunnel: "Current source K6221 VISA" -> [w6 w24 _ w58 w111 w113]
    tunnel: w1 -> [_ _ _ w56 _ _]
    frame #0 {
      n3 = flat-sequence {
        tunnel: w6 -> [w8]
        tunnel: [w9] -> w4
        tunnel: [w12] -> w7
        tunnel: w4 -> [w13]
        tunnel: w7 -> [w15]
        tunnel: w5 -> [w17]
        frame #0 {
          n4 = call "KE622x -- Set Current Range.vi"("Resource In"=w8, "Current Range In"="Current Range In") -> ("Resource Out (dupl)"=w9:refnum<visa-resource-name>)  [unwired: 11 in, 2 out]
        }
        frame #1 {
          n5 = call "KE622x -- Set Current Level.vi"("Resource In"=w13, "Current Level (A) In"=0.0 ("Set I (A)")) -> ("Resource Out (dupl)"=w12:refnum<visa-resource-name>)  [unwired: 11 in, 2 out]
        }
        frame #2 {
          n6 = call "KE622x -- Set Output State.vi"("Resource In"=w15, "Output State"=1) -> ()  [unwired: 12 in, 2 out]
        }
        frame #3 {
          n7 = Wait (ms)(milliseconds to wait=100) -> ()  [unwired: 1 out]
        }
        frame #4 {
          n8 = for {
            N: 5 ("Numeric") -> [_]
            tunnel: w17 -> [w19]
            w21 = u16 1 items=["Slow", "Med", "Fast"] ("Rate (NPLC)")
            w22 = FALSE ("Auto range?")
            n9 = call "Initialize_K2182A_VISA_PK.vi"("VISA address"=w19, "Auto range?"=TRUE, "Analog LPass\nFilter?"=w22, "DC\nFilter?"=w22, "Rate (NPLC)"=w21) -> ()  [unwired: 2 in]
          }
        }
      }
    }
    frame #1 {
      w30 = "\t"
      n10 = Concatenate Strings("file name", ".dat" ("string")) -> (w36:string)
      n11 = String To Path(string=w36) -> (path=w26:path)
      n12 = call "KE622x -- Set Voltage Limit.vi"("Resource In"=w24, "Voltage Limit (V)"="Set Compliance voltage (V)") -> ()  [unwired: 12 in, 2 out]
      n13 = Concatenate Strings("V (V)" ("string"), w30, "I (A)" ("string"), w30, "R (Ohm)" ("string"), "\r\n") -> (w37:string)
      n14 = Build Path(base path="Folder", name or relative path=w26) -> (appended path=w25:path)
      n15 = flat-sequence {
        tunnel: w25 -> [w43]
        tunnel: w37 -> [w46]
        tunnel: [w46] -> w39
        tunnel: [w45] -> w34
        tunnel: [w44] -> w38
        tunnel: w39 -> [w53]
        tunnel: w38 -> [w52]
        frame #0 {
          n16 = Open/Create/Replace File(file path (use dialog)=w43, operation (0:open)=T3."create") -> (error out=w42:errorcluster)  [unwired: 4 in, 2 out]
          n17 = Unbundle By Name(w42) -> ("status"=w40:bool)
          n18 = case shown="True" w40 {
            tunnel: [FALSE ("Yes") w50] -> w45
            tunnel: [w47 w49] -> w44
            tunnel: w43 -> [w47 w49]
            frame False {
            }
            frame True {
              n19 = call "Message to User"() -> ("Yes"=w51:bool)  [unwired: 10 in, 1 out]
              n20 = Not(x=w51) -> (.not. x?=w50:bool)
            }
          }
        }
        frame #1 {
          n21 = call <vilib>:"Write Characters To File.vi"("append to file? (new file:F)"=TRUE, "character string"=w53, "file path (dialog if empty)"=w52) -> ()  [unwired: 2 in, 1 out]
          "File path" <- w52
        }
      }
      n22 = Stop(stop? (T)=w34) -> ()
    }
    frame #2 {
      n23 = Wait (ms)(milliseconds to wait=u32 1000) -> ()  [unwired: 1 out]
    }
    frame #3 {
      n24 = for {
        N: "Total number of I-V loops" -> [_]
        tunnel: w59 -> [w63]
        tunnel: w58 -> [w62]
        tunnel: w56 -> [w60]
        n25 = for {
          tunnel: "From" -> [w70] mode=indexing
          tunnel: "To" -> [w69] mode=indexing
          tunnel: "Step" -> [w68] mode=indexing
          tunnel: w63 -> [w75]
          tunnel: w62 -> [w74]
          shift-right: [w72] -> _
          shift-left: cluster{dbl, "Field Reading":dbl}[] [] -> [w73]
          tunnel: w60 -> [w67]
          n26 = call "Build_serie_EL.vi"("end value"=w69, "increment"=w68, "start value"=w70) -> ("output array"=w71:dbl[])
          n27 = for {
            tunnel: w71 -> [w79] mode=indexing
            tunnel: w75 -> [w81]
            tunnel: w74 -> [w80]
            shift-right: [w77] -> w72
            shift-left: w73 -> [w78]
            tunnel: w67 -> [w76]
            n28 = stacked-sequence {
              tunnel: w81 -> [_ _ w95 _]
              tunnel: w80 -> [w83 _ w94 _]
              tunnel: w78 -> [_ _ w98 _]
              tunnel: w79 -> [w82 _ _ _]
              tunnel: [_ _ w97 _] -> w77
              tunnel: w76 -> [_ _ w87 _]
              frame #0 {
                n29 = call "KE622x -- Set Current Level.vi"("Resource In"=w83, "Current Level (A) In"=w82) -> ()  [unwired: 11 in, 3 out]
              }
              frame #1 {
                n30 = Wait (ms)(milliseconds to wait="wait (ms)") -> ()  [unwired: 1 out]
              }
              frame #2 {
                n31 = call <vilib>:"High Resolution Relative Seconds.vi"() -> ("relative seconds"=w86:dbl)
                n32 = Subtract(x=w86, y=w87) -> (x-y=→"Time (s)":dbl)
                n33 = for {
                  N: "Numeric Average" -> [_]
                  tunnel: [w104] -> w96 mode=indexing
                  tunnel: w95 -> [w103]
                  tunnel: w94 -> [w102]
                  tunnel: [w101] -> w93 mode=indexing
                  n34 = call "Get-V_K2182A_VISA_EL.vi"("VISA K2182A"=w103) -> ("V (V)"=w104:dbl)  [unwired: 2 in, 2 out]
                  n35 = call "KE622x -- Get Current Level.vi"("Resource In"=w102) -> ("Current Level (A)"=w101:T4)  [unwired: 12 in, 2 out]
                }
                n36 = call "Array averaging_PK.vi"("Number averaging"="Numeric Average", "numeric array"=w96) -> ("Average value"=w90:dbl)  [unwired: 9 in]
                "Vmeas (V)" <- w90
                n37 = call "Array averaging_PK.vi"("Number averaging"="Numeric Average", "numeric array"=w93) -> ("Average value"=w89:dbl)  [unwired: 9 in]
                "Iset (A)" <- w89
                n38 = Divide(x=w90, y=w89) -> (x/y=→"Resistance (ohm)":dbl)
                n39 = Divide(x=w90, y=w89) -> (x/y=w91:dbl)
                n40 = Bundle("Average value"=w89, "Average value"=w90) -> (w99:T5)  [unwired: 1 in]
                n41 = Build Array (concatenate)(w98, w99) -> (w97:T6)
                "I vs V" <- w97
                n42 = Build Array (concatenate)(w96, w89, w91) -> (→"data":dbl[])
              }
              frame #3 {
                n43 = local read "data"() -> (w105:dbl[])
                n44 = local read "File path"() -> (w107:path)
                n45 = Array To Spreadsheet String(array=w105, 3:"%e" ("format string")) -> (spreadsheet string=w108:string)  [unwired: 1 in]
                n46 = call <vilib>:"Write Characters To File.vi"("append to file? (new file:F)"=TRUE, "character string"=w108, "file path (dialog if empty)"=w107) -> ()  [unwired: 2 in, 1 out]
              }
            }
          }
        }
      }
    }
    frame #4 {
      n47 = call "KE622x -- Set Voltage Limit.vi"("Resource In"=w111, "Voltage Limit (V)"=0.1 ("Set Compliance voltage (V)")) -> ()  [unwired: 12 in, 2 out]
    }
    frame #5 {
      n48 = flat-sequence {
        tunnel: w113 -> [w116]
        tunnel: [w114] -> w112
        tunnel: w112 -> [w118]
        frame #0 {
          n49 = call "KE622x -- Set Current Level.vi"("Resource In"=w116, "Current Level (A) In"=0.0 ("Set I (A)")) -> ("Resource Out (dupl)"=w114:refnum<visa-resource-name>)  [unwired: 11 in, 2 out]
        }
        frame #1 {
          n50 = call "KE622x -- Set Output State.vi"("Resource In"=w118, "Output State"=0) -> ()  [unwired: 12 in, 2 out]
        }
      }
    }
  }
